vi "Get Target Current.vi"(0 "VISA resource name":refnum<visa-resource-name>, 1 "error in":T1) -> (2 "VISA resource name out":refnum<visa-resource-name>, 3 "Target Current (A)":dbl format="%.3f", 4 "error out":T1)   [LabVIEW 2019]
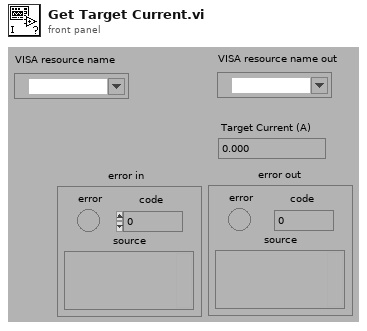
[diagram p1: front panel]
types:
  T1 = cluster{"error":bool, "code":i32, "source":string}
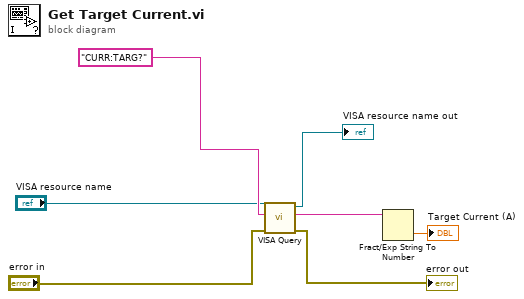
[diagram p0: block diagram]
diagram:
  n1 = call "VISA Query.vi"("error in (no error)"="error in", "Command"="CURR:TARG?", "VISA resource name"="VISA resource name") -> ("error out"=→"error out":errorcluster, "Response"=w3:string, "VISA resource name out"=→"VISA resource name out":refnum<visa-resource-name>)  [unwired: 4 in, 2 out]
  n2 = Fract/Exp String To Number(string=w3) -> (number=→"Target Current (A)":dbl)  [unwired: 3 in, 1 out]
